vi "Rotation3d_RotateBy.vi"(9 "other Rotation3d":T1={"Q_quaternion"={"R"=1.0, "V"=[0.0, 0.0, 0.0]}}, 11 "in Rotation3d":T1={"Q_quaternion"={"R"=1.0, "V"=[0.0, 0.0, 0.0]}}) -> (3 "out Rotation3d":T1={"Q_quaternion"={"R"=1.0, "V"=[0.0, 0.0, 0.0]}})   [LabVIEW 2019, in "Trajectory_Library.lvlib"]
doc: "Adds the new rotation to the current rotation using a rotation matrix.\n\nThe matrix multiplication is as follows:\n [cos_new] [other.cos, -other.sin][cos]\n [sin_new] = [other.sin, other.cos][sin]\n value_new = atan2(cos_new, sin_new)\n\nThis is the same as Plus.\n\nParameters:\n - IN ROTATION - This ROTATION data structure\n - OTHER ROTATION - The rotation to rotate by\n\nReturns:\n - OUT ROTATION - The new rotated Rotation2d."
uses:
  Trajectory_Library.lvlib
  ROTATION3D.ctl
  QUATERNION.ctl
  Quaternion_Normalize.vi
  Quaternion_Get_LVQuat.vi
  Quaternion_New_LVQuat.vi
  Quaternion_Equals.vi
  Quaternion_New_Default.vi
  <vilib>/robotics/Kinematics/Multiply Quaternions.vi
  <vilib>/robotics/Kinematics/Multiply Quaternion by Quaternion.vi
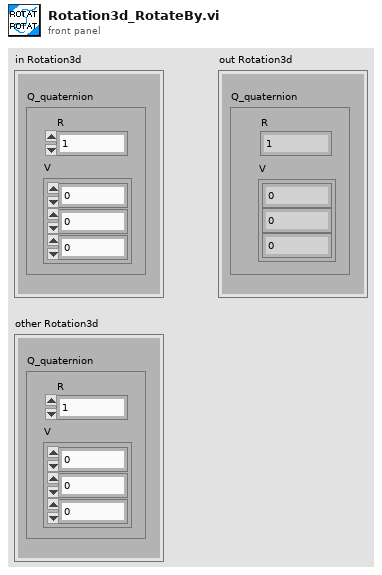
[diagram p1: front panel]
types:
  T1 = typedef "Trajectory_Library.lvlib/ROTATION3D.ctl" = cluster{"Q_quaternion":T2}
  T2 = typedef "Trajectory_Library.lvlib/QUATERNION.ctl" = cluster{"R":dbl, "V":dbl[]}
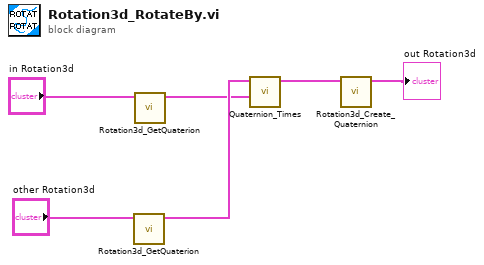
[diagram p0: block diagram]
diagram:
  n1 = call "Rotation3d_GetQuaterion.vi"("in Rotation3d"="other Rotation3d") -> ("out Quaterion"=w3:T2)  [unwired: 10 in]
  n2 = call "Rotation3d_GetQuaterion.vi"("in Rotation3d"="in Rotation3d") -> ("out Quaterion"=w1:T2)  [unwired: 10 in]
  n3 = call "Quaternion_Times.vi"("Other Quaternion"=w1, "Quaternion"=w3) -> ("Times"=w5:T2)  [unwired: 6 in, 3 out]
  n4 = call "Rotation3d_Create_Quaternion.vi"("Quaternion"=w5) -> ("Rotation3d"=→"out Rotation3d":T1)  [unwired: 10 in]
